vi "old_HWGlobalsToObject.vi"(7 "Select Layout":refnum<vi>, 8 "error in (no error)":errorcluster, 9 "Trigger Lines":u16[](array[numeric]), 10 "Name":string, 11 "Pulseblaster in":refnum<class "Pulseblaster.lvclass">) -> (0 "error out":errorcluster, 3 "Pulseblaster out":refnum<class "Pulseblaster.lvclass">)   [LabVIEW 2013, in "Pulseblaster.lvclass"]
doc: "Set device name and denote which trigger lines are being used.\nThis information is used to initialize the device and it's \"appearance\" Column array."
uses:
  Pulseblaster.lvclass
  Pulseblaster.lvclass/Pulseblaster.ctl
panel:
  in  "Definitions":T1={"External MemorySize"=32768, "Internal Memory Size"=512, "Overhead Ticks"=3, "Min Delay Loops"=3, "Loop Count Correction"=1, "Long Delay Loop Count Correction"=2, "Min Instruction Ticks"=6, "Long Delay Ticks"=4294967295, "Clock Period (s)"=1e-08, "Overhead Time (s)"=3e-08, "Min Instruction Cycle Time (s)"=9e-08, "Long Delay Time (s) "=42.94967298} {"Long Delay Time (s)" format="%.8p"; "Min Instruction Cycle Time (s)" format="%.0p"; "Overhead Time (s)" format="%.0p"; "Clock Period (s)" format="%.0p"; "Long Delay Ticks" format="%.0x"}
  # "(Period*Long D Ticks)+Overhead time"
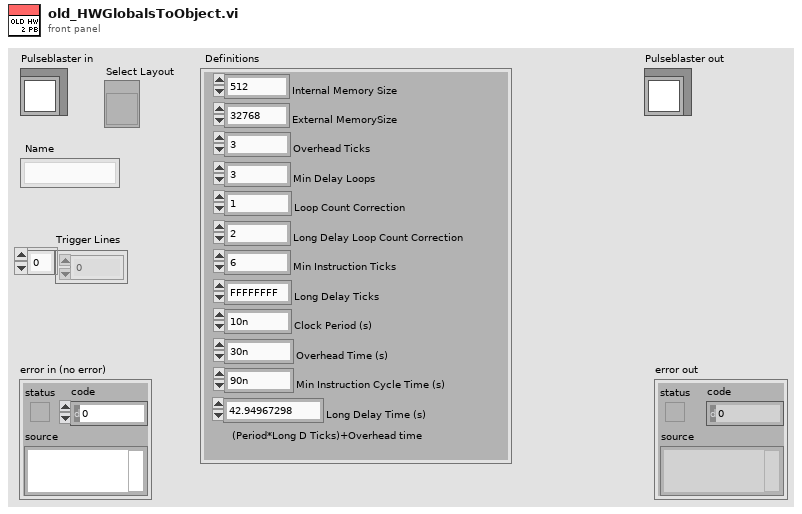
[diagram p1: front panel]
types:
  T1 = cluster{"External MemorySize":u16, "Internal Memory Size":u16, "Overhead Ticks":u8, "Min Delay Loops":u8, "Loop Count Correction":u8, "Long Delay Loop Count Correction":u8, "Min Instruction Ticks":u8, "Long Delay Ticks":u64, "Clock Period (s)":dbl, "Overhead Time (s)":dbl, "Min Instruction Cycle Time (s)":dbl, "Long Delay Time (s) ":dbl}
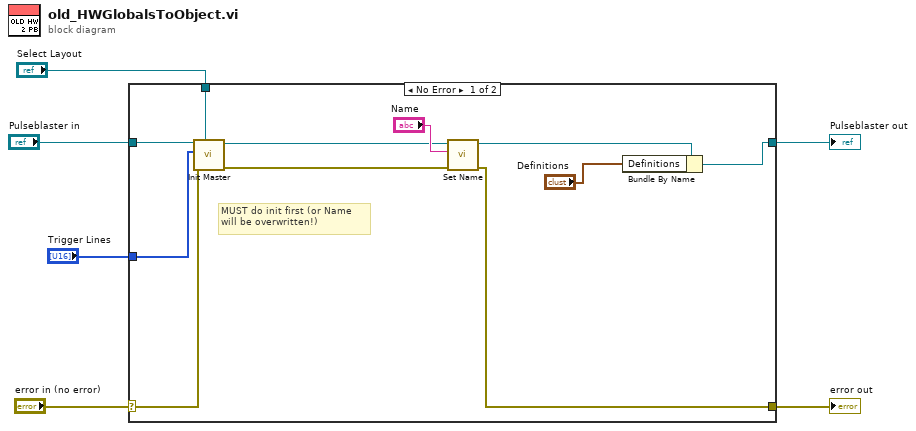
[diagram p0: block diagram]
diagram:
  n1 = case shown="No Error" "error in (no error)" {
    selector: "error in (no error)" -> [w12 w19]
    tunnel: [w9 w19] -> w5
    tunnel: [w16 w18] -> w3
    tunnel: "Pulseblaster in" -> [w7 w18]
    tunnel: "Trigger Lines" -> [w14 _]
    tunnel: "Select Layout" -> [w13 _]
    frame No Error {
      # "MUST do init first (or Name \nwill be overwritten!)"
      n2 = call-dynamic "Init Master.vi"("Select Layout"=w13, "error in (no error)"=w12, "Trigger Lines"=w14, "Pulseblaster in"=w7) -> ("error out"=w11:errorcluster, "Pulseblaster out"=w10:refnum<class "Pulseblaster.lvclass">)  [unwired: 6 in]
      n3 = call-dynamic "Set Name.vi"("error in (no error)"=w11, "Name"="Name", "Device in"=w10) -> ("error out"=w9:errorcluster, "Device out"=w8:refnum<class "Pulseblaster.lvclass">)  [unwired: 7 in]
      n4 = Bundle By Name(cluster=w8, "Definitions"="Definitions") -> (w16:refnum<class "Pulseblaster.lvclass">)
    }
    frame Error {
    }
  }
  "error out" <- w5
  "Pulseblaster out" <- w3
